vi "m300Allocation.vi"() -> ()   [LabVIEW 2012]
uses:
  <vilib>/Utility/NIReport.llb/NI_report.lvclass
  <vilib>/addons/database/Connection.llb/DB Tools Open Connec (Path).vi
  <vilib>/addons/database/Connection.llb/Conn Execute.vi
  <vilib>/addons/database/Recordset.llb/Rec Fetch Recordset Data (R).vi
  <vilib>/addons/database/Recordset.llb/Rec Destroy - Connection.vi
  <vilib>/Utility/NIReport.llb/Append Text Table to Report (wrap).vi
  <vilib>/addons/database/_DB Variant To Data/Database Variant To Data.xnode
  <vilib>/addons/database/NI_Database_API.lvlib
  <vilib>/Utility/NIReport.llb/Excel/NI_Excel.lvclass
  <vilib>/addons/_office/NI_ReportGenerationToolkit.lvlib
panel:
  out "Array":string[][](array[string])
  in  "Report Template":path=path "O:/Monitor/Report/M300Allocation.xls"
  out "error out 2":errorcluster
  in  "Table Control":string[][](table)
  out "error out 3":errorcluster
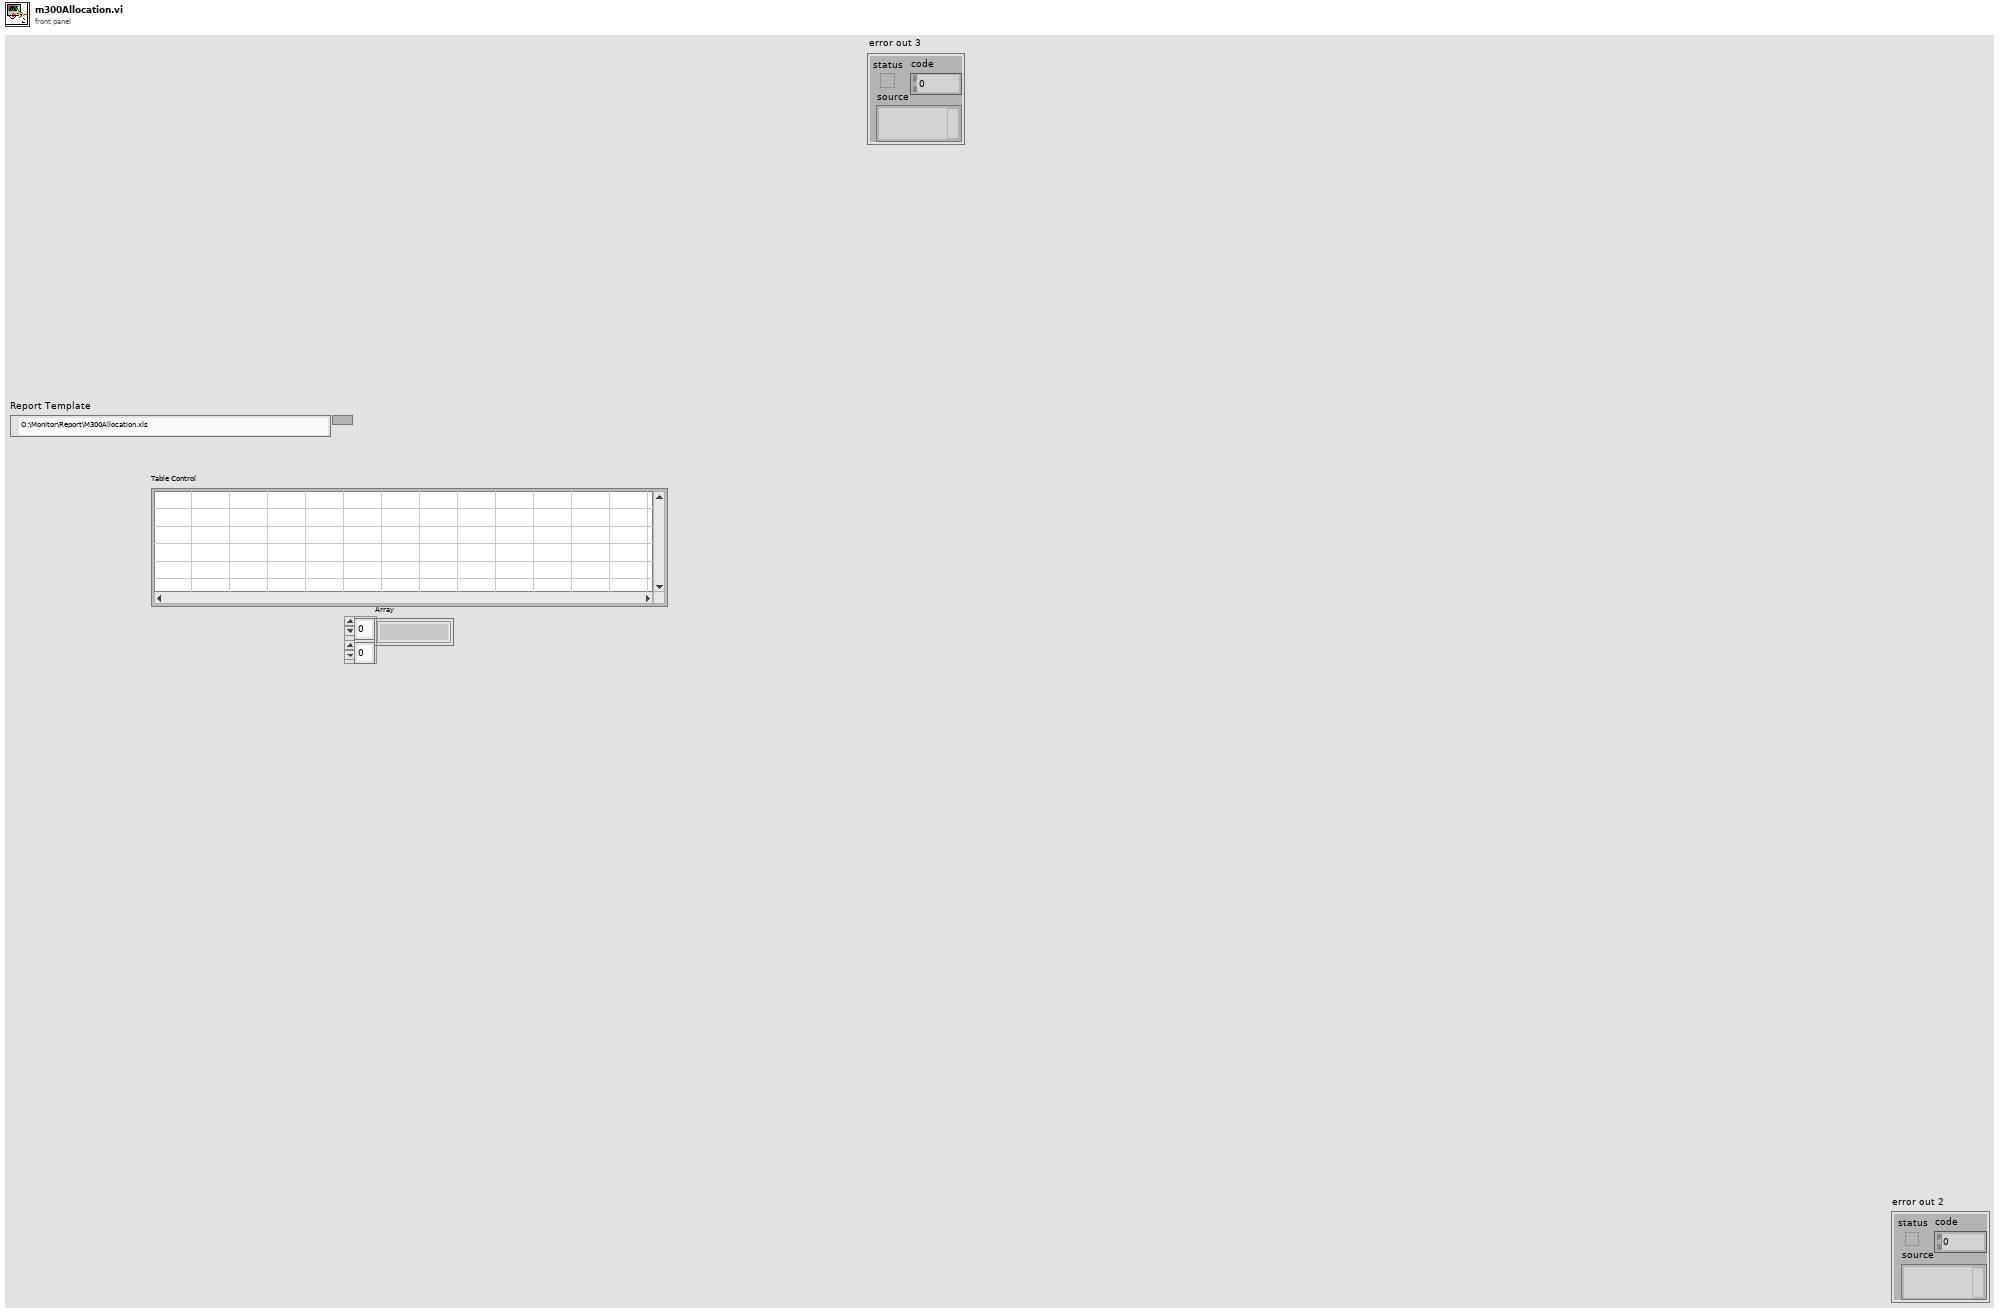
[diagram p1: front panel]
types:
  T1 = typedef "NI_Database_API.lvlib/Conn ObjectReference.ctl" = refnum<k1>
  T2 = typedef "NI_Database_API.lvlib/Rec ObjectReference.ctl" = refnum<k1>
  T3 = enum16{"Standard Report", "HTML", "Word", "Excel"}
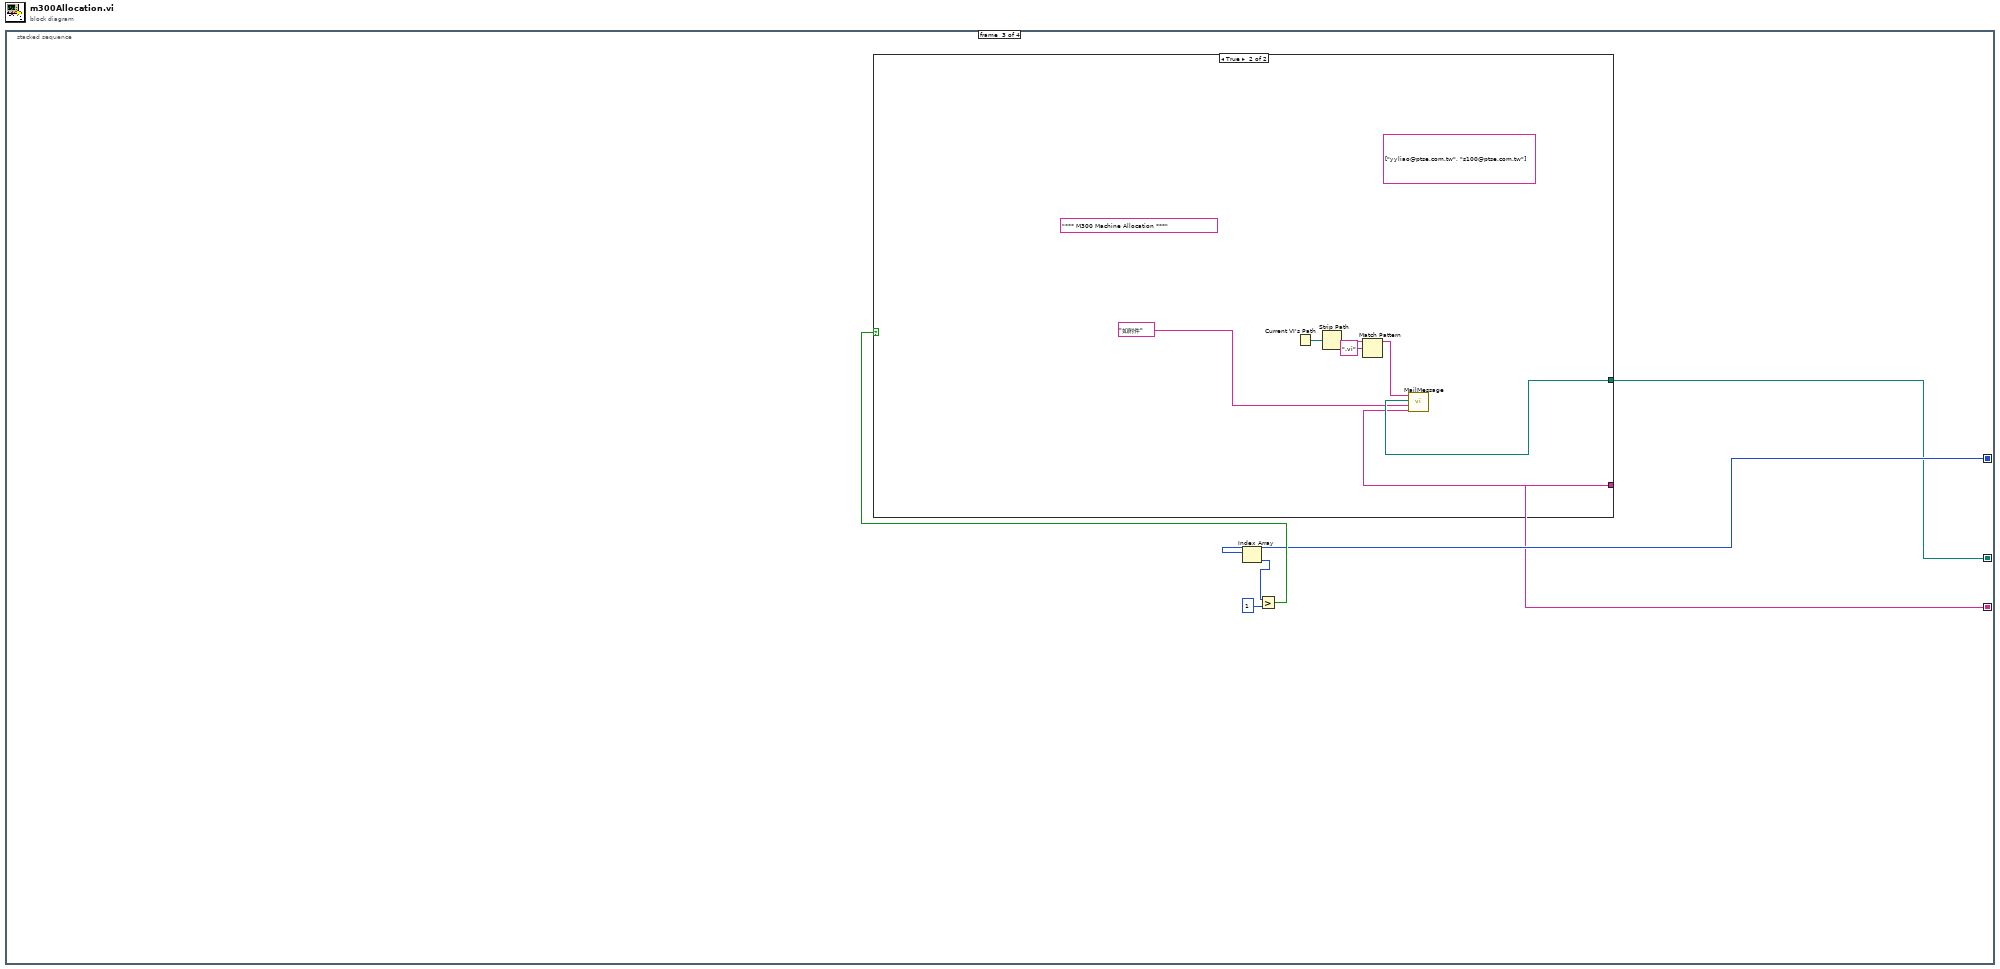
[diagram p0: block diagram]
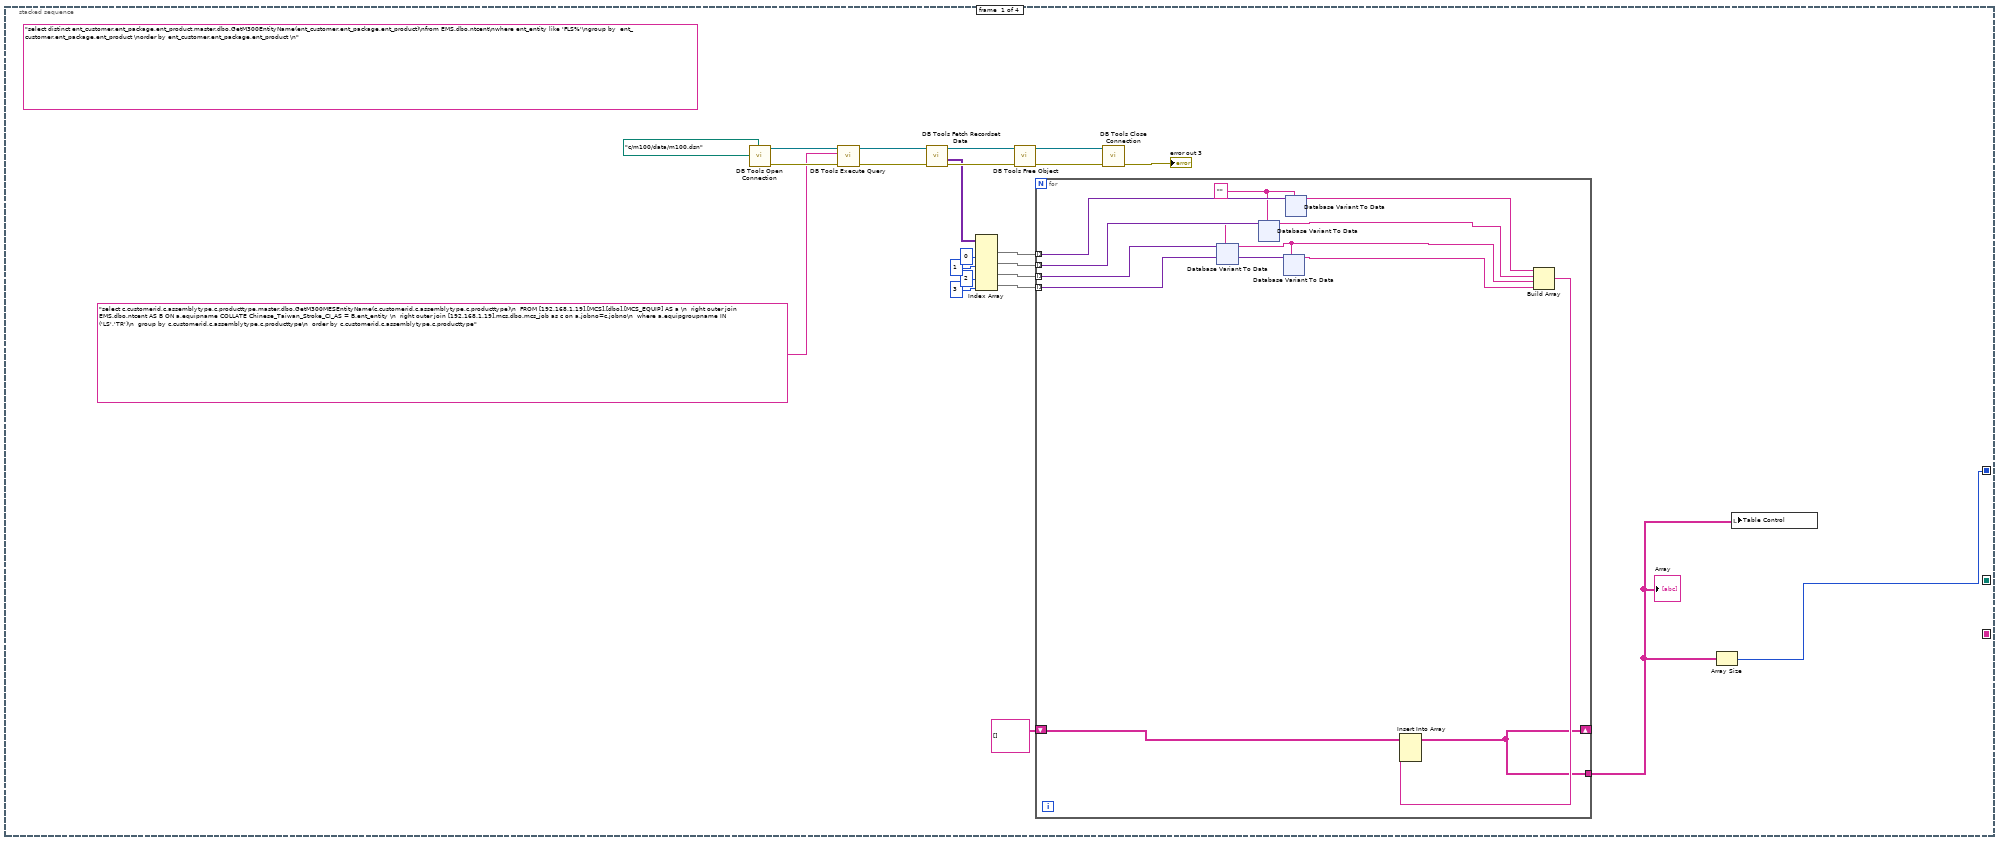
[diagram p2: hidden frame]
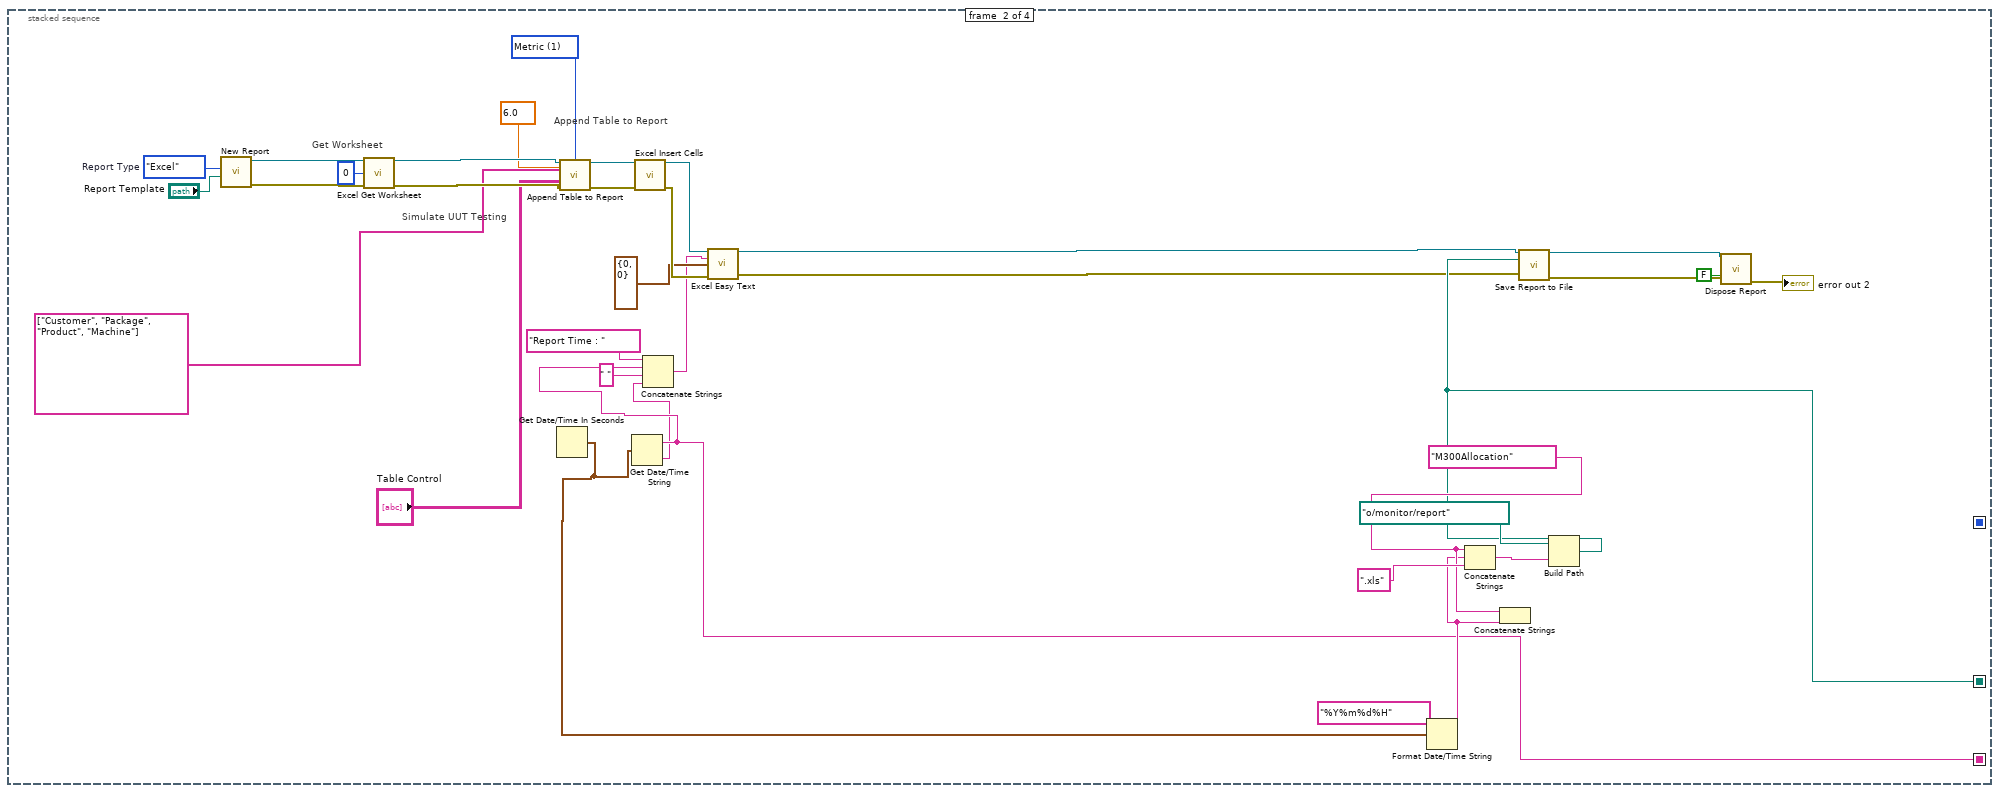
[diagram p3: hidden frame]
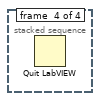
[diagram p5: hidden frame]
diagram:
  n1 = stacked-sequence {
    seq-local: [w2 _ _ _] -> [_ _ w201 _]
    seq-local: [_ w173 _ _] -> [_ _ w200 _]
    seq-local: [_ w170 _ _] -> [_ _ w199 _]
    frame #0 {
      (unwired) "select distinct ent_customer,ent_package,ent_product,master.dbo.GetM300EntityName(ent_customer,ent_package,ent_product)\nfrom EMS.dbo.ntcent\nwhere ent_entity like 'FLS%'\ngroup by  ent_customer,ent_package,ent_product \norder by ent_customer,ent_package,ent_product \n" ("SQL query")
      n2 = call-poly <vilib>:"DB Tools Open Connection.vi"("connection information"=path "c:/m100/data/m100.dsn") -> ("error out"=w18:errorcluster, "connection reference"=w22:T1)  [unwired: 7 in]
      n3 = call-poly <vilib>:"DB Tools Execute Query.vi"("error in (no error)"=w18, "SQL query"="select c.customerid,c.assemblytype,c.producttype,master.dbo.GetM300MESEntityName(c.customerid,c.assemblytype,c.producttype)\n  FROM [192.168.1.19].[MCS].[dbo].[MCS_EQUIP] AS a \n  right outer join EMS.dbo.ntcent AS B ON a.equipname COLLATE Chinese_Taiwan_Stroke_CI_AS = B.ent_entity \n  right outer join [192.168.1.19].mcs.dbo.mcs_job as c on a.jobno=c.jobno\n  where a.equipgroupname IN ('LS','TR')\n  group by c.customerid,c.assemblytype,c.producttype\n  order by c.customerid,c.assemblytype,c.producttype", "connection reference"=w22) -> ("error out"=w17:errorcluster, "recordset reference"=w21:T2)  [unwired: 5 in]
      n4 = call-poly <vilib>:"DB Tools Fetch Recordset Data.vi"("error in (no error)"=w17, "recordset reference"=w21) -> ("error out"=w16:errorcluster, "recordset data"=w5:variant[][], "recordset reference out"=w20:T2)  [unwired: 3 in]
      n5 = Index Array(array=w5, index (col) #1=0 ("disabled index (col)"), index (col) #2=1 ("index (col)"), index (col) #3=2 ("index (col)"), index (col) #4=3 ("index (col)")) -> (element #1=w9:variant[], element #2=w8:variant[], element #3=w7:variant[], element #4=w6:variant[])  [unwired: 4 in]
      n6 = call-poly <vilib>:"DB Tools Free Object.vi"("error in (no error)"=w16, "recordset reference"=w20) -> ("error out"=w15:errorcluster, "connection reference"=w19:T1)  [unwired: 8 in]
      n7 = for {
        tunnel: w9 -> [w35] mode=indexing
        tunnel: w8 -> [w34] mode=indexing
        tunnel: w7 -> [w33] mode=indexing
        tunnel: w6 -> [w32] mode=indexing
        tunnel: [w29] -> w3
        shift-right: [w29] -> _
        shift-left: string[][] [] -> [w28]
        w25 = ""
        n8 = xnode "Database Variant To Data"("database variant"=w33, "type"=w25) -> ("data"=w24:string)  [unwired: 1 in, 1 out]
        n9 = xnode "Database Variant To Data"("database variant"=w34, "type"=w25) -> ("data"=w27:string)  [unwired: 1 in, 1 out]
        n10 = xnode "Database Variant To Data"("database variant"=w32, "type"=w24) -> ("data"=w26:string)  [unwired: 1 in, 1 out]
        n11 = xnode "Database Variant To Data"("database variant"=w35, "type"=w25) -> ("data"=w31:string)  [unwired: 1 in, 1 out]
        n12 = Build Array(w31, w27, w24, w26) -> (w30:string[])
        n13 = Insert Into Array(array=w28, new element=w30) -> (w29:string[][])  [unwired: 2 in]
      }
      "Array" <- w3
      n14 = call <vilib>:"DB Tools Close Connection.vi"("error in (no error)"=w15, "connection reference"=w19) -> ("error out"=→"error out 3":errorcluster)  [unwired: 5 in]
      n15 = Array Size(array=w3) -> (size(s)=w2:i32[])
      n16 = local write "Table Control"(w3) -> ()
    }
    frame #1 {
      w177 = u16 1 items=["US", "Metric", "Default"] ("measurement system")
      w178 = "M300Allocation"
      w198 = T3."Excel"  # Report Type
      # "Simulate UUT Testing"
      # "Append Table to Report"
      # "Get Worksheet"
      n17 = call <vilib>:"New Report.vi"("report type"=w198, "template (empty)"="Report Template") -> ("report out"=w194:refnum<class "NI_report.lvclass">, "error out"=w193:errorcluster)  [unwired: 12 in]
      n18 = call <vilib>:"Excel Get Worksheet.vi"("report in"=w194, "worksheet index (0)"=0, "error in (no error)"=w193) -> ("report out"=w183:refnum<class "NI_report.lvclass">, "error out"=w182:errorcluster)  [unwired: 11 in]
      n19 = Get Date/Time In Seconds() -> (seconds since 1Jan1904=w168:timestamp)
      n20 = call-poly <vilib>:"Append Table to Report.vi"("report in"=w183, "column width (1)"=6.0, "measurement system"=w177, "column headers"=string[] ["Customer", "Package", "Product", "Machine"] ("row headers"), "text data"="Table Control", "error in (no error)"=w182) -> ("report out"=w196:refnum<class "NI_report.lvclass">, "error out"=w195:errorcluster)  [unwired: 6 in, 2 out]
      n21 = Get Date/Time String(seconds (now)=w168) -> (date string=w170:string, time string=w169:string)  [unwired: 2 in]
      n22 = call <vilib>:"Excel Insert Cells.vi"("report in"=w196, "error in (no error)"=w195) -> ("report out"=w190:refnum<class "NI_report.lvclass">, "error out"=w189:errorcluster)  [unwired: 12 in]
      n23 = Concatenate Strings("Report Time : " ("string"), w170, " " ("string"), w169) -> (w186:string)
      n24 = call <vilib>:"Excel Easy Text.vi"("report in"=w190, "text"=w186, "start (-1, -1)"=cluster{"row":i32, "column":i32} {"row"=0, "column"=0} ("end (-1, -1)"), "error in (no error)"=w189) -> ("report out"=w166:refnum<class "NI_report.lvclass">, "error out"=w165:errorcluster)  [unwired: 7 in, 3 out]
      n25 = Format Date/Time String(time format string (%c)="%Y%m%d%H", seconds (now)=w168) -> (date/time string=w175:string)  [unwired: 1 in]
      n26 = Concatenate Strings(w178, w175, ".xls" ("string")) -> (w179:string)
      n27 = Concatenate Strings(w178, w175) -> ()  [unwired: 1 out]
      n28 = Build Path(base path=path "o:/monitor/report", name or relative path=w179) -> (appended path=w173:path)
      n29 = call-dynamic "Save Report to File.vi"("report in"=w166, "report file path"=w173, "error in (no error)"=w165) -> ("report out"=w185:refnum<class "NI_report.lvclass">, "error out"=w184:errorcluster)  [unwired: 11 in]
      n30 = call-dynamic "Dispose Report.vi"("report in"=w185, "save changes? (F)"=FALSE, "error in (no error)"=w184) -> ("error out"=→"error out 2":errorcluster)  [unwired: 12 in]
    }
    frame #2 {
      n31 = Index Array(array=w201) -> (element=w204:i32)  [unwired: 1 in]
      n32 = Greater?(x=w204, y=1) -> (0:w202:bool)
      n33 = case shown="True" w202 {
        tunnel: w200 -> [_ w207]
        tunnel: w199 -> [_ w206]
        frame False {
        }
        frame True {
          (unwired) string[] ["yyliao@ptse.com.tw", "s100@ptse.com.tw"] ("recipients")
          (unwired) "*** M300 Machine Allocation ***" ("subject ([No Subject])")
          n34 = Current VI's Path() -> (path=w211:path)
          n35 = Strip Path(path=w211) -> (name=w210:string)  [unwired: 1 out]
          n36 = Match Pattern(string=w210, regular expression=".vi") -> (before substring=w208:string)  [unwired: 1 in, 3 out]
          n37 = call "MailMessage.vi"("AddSubject"=w206, "message"="如附件", "file path"=w207, "program"=w208) -> ()  [unwired: 8 in]
        }
      }
    }
    frame #3 {
      n38 = Quit LabVIEW() -> ()  [unwired: 1 in]
    }
  }
